vi "stage_abort.vi"(8 "error in (no error)":errorcluster, 10 "Stage Name":string, 11 "newport_xps in":refnum<class "newport_xps.lvclass">) -> (0 "error out":errorcluster, 3 "newport_xps out":refnum<class "newport_xps.lvclass">)   [LabVIEW 2015, in "newport_xps.lvclass"]
uses:
  newport_xps.lvclass
  newport_xps.lvclass/newport_xps.ctl
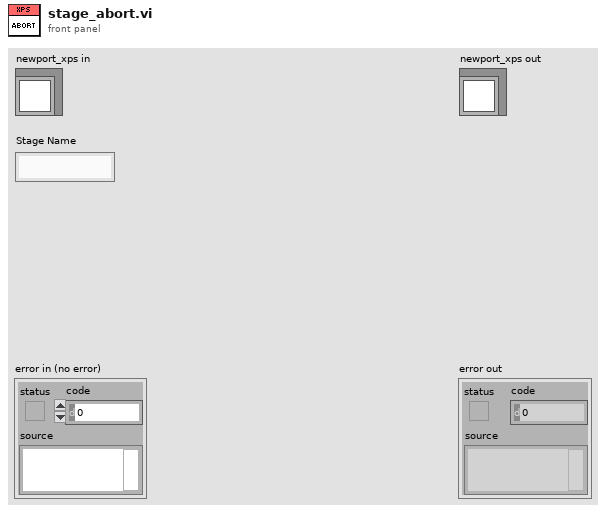
[diagram p1: front panel]
types:
  T1 = cluster{"connection TCP":refnum<k5>, "LogTo File":bool, "Log File refnum":refnum<file>, "no error if error log":bool}
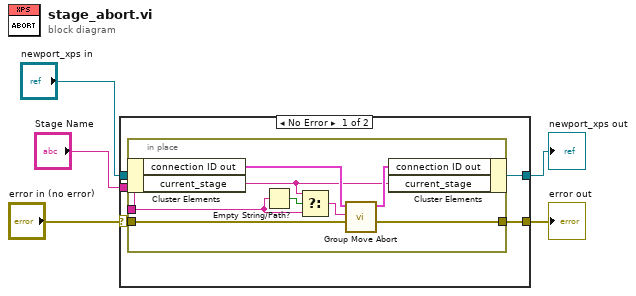
[diagram p0: block diagram]
diagram:
  n1 = case shown="No Error" "error in (no error)" {
    selector: "error in (no error)" -> [w8 w19]
    tunnel: "newport_xps in" -> [w10 w20]
    tunnel: "Stage Name" -> [w9 _]
    tunnel: [w7 w19] -> w2
    tunnel: [w6 w20] -> w1
    frame No Error {
      n2 = in-place {
        in-place-border: w9 -> [w15]
        in-place-border: w8 -> [w12]
        in-place-border: [w11] -> w7
        n3 = in-place-cluster #1(w10) -> ("connection ID out"=w18:T1, "current_stage"=w13:string)
        n4 = Empty String/Path?(string/path=w15) -> (empty?=w16:bool)
        n5 = Select(t=w13, s=w16, f=w15) -> (s? t:f=w14:string)
        n6 = call "Group Move Abort.vi"("XPS error in (no error)"=w12, "Group Name (250 c max)"=w14, "connection ID in"=w18) -> ("XPS error out"=w11:errorcluster, "connection ID out"=w17:T1)  [unwired: 6 in, 1 out]
        n7 = in-place-cluster #1("connection ID out"=w17, "current_stage"=w13) -> (w6:refnum<class "newport_xps.lvclass">)
      }
    }
    frame Error {
    }
  }
  "error out" <- w2
  "newport_xps out" <- w1
